vi "Create Pattern Script(Data_4W).vi"(7 "DataType":T1, 8 "error in (no error)":errorcluster, 11 "Data":u16) -> (0 "error out":errorcluster, 3 "String":string)   [LabVIEW 2018, in "SPI_Frame_Root.lvclass"]
uses:
  SPI_Frame_Root.lvclass
  DataType.ctl
  Classes/BML_Frame_Root/BML_Frame_Root.lvclass
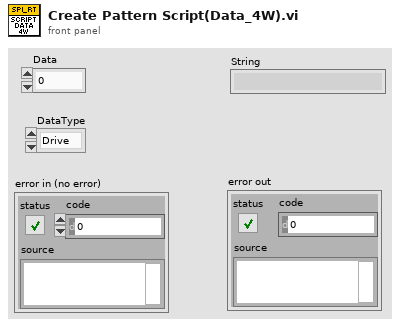
[diagram p1: front panel]
types:
  T1 = typedef "SPI_Frame_Root.lvclass/DataType.ctl" = enum16{"Drive", "Compare", "Read"}
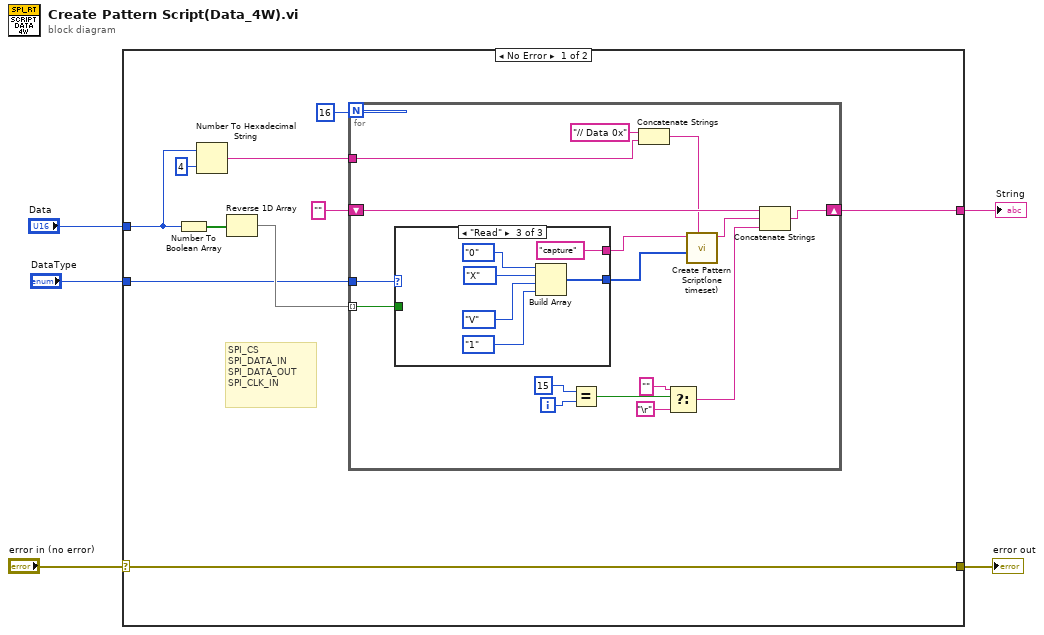
[diagram p0: block diagram]
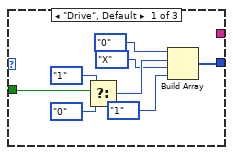
[diagram p2: hidden frame]
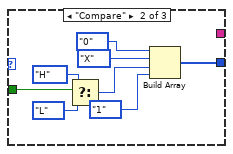
[diagram p3: hidden frame]
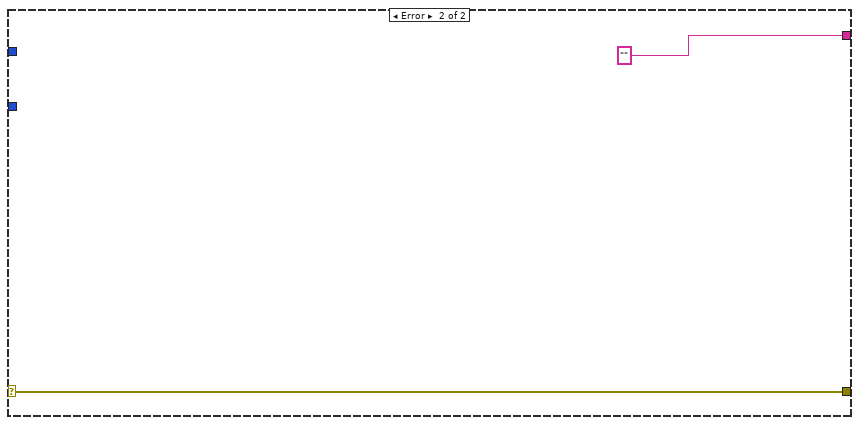
[diagram p4: hidden frame]
diagram:
  n1 = case shown="No Error" "error in (no error)" {
    selector: "error in (no error)" -> [w15 w54]
    tunnel: [w6 ""] -> w4
    tunnel: [w15 w54] -> w3
    tunnel: "Data" -> [w9 _]
    tunnel: "DataType" -> [w7 _]
    frame No Error {
      # "SPI_CS\nSPI_DATA_IN\nSPI_DATA_OUT\nSPI_CLK_IN"
      n2 = Number To Boolean Array(number=w9) -> (Boolean array=w11:bool[])
      n3 = Number To Hexadecimal String(1:i16 4 ("width (-)"), 2:w9) -> (0:w12:string)
      n4 = Reverse 1D Array(array=w11) -> (reversed array=w8:bool[])
      n5 = for {
        N: 16 -> [_]
        shift-right: [w26] -> w6
        shift-left: "" -> [w25]
        tunnel: w12 -> [w21]
        tunnel: w8 -> [w18] mode=indexing
        tunnel: w7 -> [w19]
        i -> [w31]
        n6 = case shown="\"Read\"" w19 {
          tunnel: w18 -> [w35 w44 _]
          tunnel: [w32 w40 w50] -> w17
          tunnel: [_ _ "capture" ("opcode")] -> w16
          frame "Drive", Default {
            n7 = Select(t=enum16{"0", "1", "L", "H", "X", "V", "D", "M"}."1" ("PinState"), s=w35, f=enum16{"0", "1", "L", "H", "X", "V", "D", "M"}."0") -> (s? t:f=w34:enum16{"0", "1", "L", "H", "X", "V", "D", "M"})
            n8 = Build Array(enum16{"0", "1", "L", "H", "X", "V", "D", "M"}."0" ("PinState"), w34, enum16{"0", "1", "L", "H", "X", "V", "D", "M"}."X" ("element"), enum16{"0", "1", "L", "H", "X", "V", "D", "M"}."1" ("element")) -> (w32:enum16{"0", "1", "L", "H", "X", "V", "D", "M"}[])
          }
          frame "Compare" {
            n9 = Select(t=enum16{"0", "1", "L", "H", "X", "V", "D", "M"}."H" ("PinState"), s=w44, f=enum16{"0", "1", "L", "H", "X", "V", "D", "M"}."L") -> (s? t:f=w43:enum16{"0", "1", "L", "H", "X", "V", "D", "M"})
            n10 = Build Array(enum16{"0", "1", "L", "H", "X", "V", "D", "M"}."0" ("PinState"), enum16{"0", "1", "L", "H", "X", "V", "D", "M"}."X" ("element"), w43, enum16{"0", "1", "L", "H", "X", "V", "D", "M"}."1" ("element")) -> (w40:enum16{"0", "1", "L", "H", "X", "V", "D", "M"}[])
          }
          frame "Read" {
            n11 = Build Array(enum16{"0", "1", "L", "H", "X", "V", "D", "M"}."0" ("PinState"), enum16{"0", "1", "L", "H", "X", "V", "D", "M"}."X" ("element"), enum16{"0", "1", "L", "H", "X", "V", "D", "M"}."V" ("element"), enum16{"0", "1", "L", "H", "X", "V", "D", "M"}."1" ("element")) -> (w50:enum16{"0", "1", "L", "H", "X", "V", "D", "M"}[])
          }
        }
        n12 = Equal?(x=15, y=w31) -> (x = y?=w29:bool)
        n13 = Concatenate Strings("// Data 0x" ("string"), w21) -> (w20:string)
        n14 = Select(t="", s=w29, f="\r") -> (s? t:f=w24:string)
        n15 = call "Create Pattern Script(one timeset).vi"("Notes"=w20, "PinState"=w17, "opcode"=w16) -> ("string out"=w23:string)  [unwired: 8 in]
        n16 = Concatenate Strings(w25, w23, w24) -> (w26:string)
      }
    }
    frame Error {
    }
  }
  "String" <- w4
  "error out" <- w3
